vi "ATF Storage-RT_DAQ.vi"(8 "error in":errorcluster, 11 "Data FIFO Ref":T1) -> (0 "error out":errorcluster)   [LabVIEW 2022 SP3]
uses:
  RT Support/ATF Storage-RT_Global_R.vi
  RT Controls/ATF Storage-Data FIFO.ctl
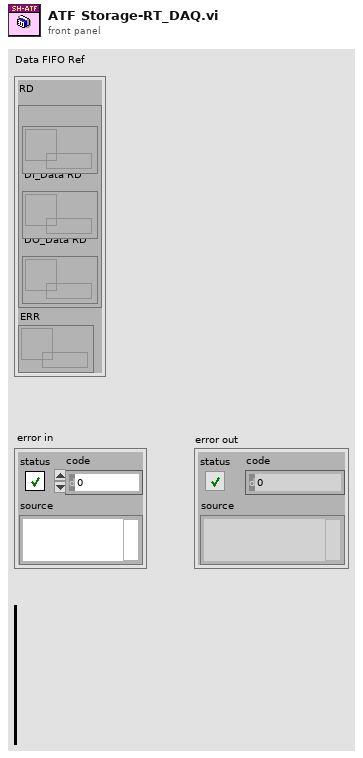
[diagram p1: front panel]
types:
  T1 = typedef "ATF Storage-Data FIFO.ctl" = cluster{"RD":cluster{"AI_V_Data RD":refnum<queue>, "DI_Data RD":refnum<queue>, "DO_Data RD":refnum<queue>}, "ERR":refnum<queue>}
  T2 = enum16{"Initialize", "Create Task", "Start", "Acquire", "Stop", "Exit"}
  T3 = cluster{"AI_Task":refnum<k21>, "AO_Task":refnum<k21>, "DI_Task":refnum<k21>, "DO_Task":refnum<k21>, "ACC_Task":refnum<k21>, "TC_Task":refnum<k21>, "AI_V_Task":refnum<k21>, " FIFO Ref":T1, "Config":cluster{"AO config":cluster{"Channel_Name":string, "Channel_Number":string, "Default_Value":dbl, "Units":string}[], "AI config":cluster{"Channel_Name":string, "Channel_Number":string, "Pre_Scale_min":dbl, "Pre_Scale_max":dbl, "Sensor_min":dbl, "Sensor_max":dbl, "Units":string}[], "DI config":cluster{"Channel_Name":string, "Channel_Number":string, "Default_Value":bool, "DI invert?":bool}[], "DO config":cluster{"Channel_Name":string, "Channel_Number":string, "Default_Value":bool, "DO invert?":bool}[], "TC config":cluster{"Channel_Name":string, "Channel_Number":string, "Pre_Scale_min":dbl, "Pre_Scale_max":dbl, "units":i32, " type":i32}[], "ACC config":cluster{"Channel_Name":string, "Channel_Number":string, "Pre_Scale_min":dbl, "Pre_Scale_max":dbl, "Terminal configuration":i32, "Sensitivity":dbl, "Sensitivity units":i32}[], "SG config":cluster{"Channel_Name":string, "Channel_Number":string, "Pre_Scale_min":dbl, "Pre_Scale_max":dbl}[], "Strain Gauge Settings":cluster{"poisson ratio":dbl, "nominal gage resistance":dbl, "gage factor":dbl}, "Bridge Settings":cluster{"voltage excitation value":dbl, "voltage excitation source":i32, "initial bridge voltage":dbl, "lead wire resistance":dbl, "strain configuration":i32}, "Sample Rate":cluster{"AI Sample Rate":dbl[], "AO Sample Rate":dbl[], "DI Sample Rate":dbl[], "TC Sample Rate":dbl[], "DO Sample Rate":dbl[], "SG Sample Rate":dbl[], "ACC Sample Rate":dbl[]}}}
  T4 = cluster{"Start DAQ":bool, "Stop DAQ":bool, "RT Stop":bool, "RT Exit":bool, "Start Seq":bool}
  T5 = cluster{"AO config":cluster{"Channel_Name":string, "Channel_Number":string, "Default_Value":dbl, "Units":string}[], "AI config":cluster{"Channel_Name":string, "Channel_Number":string, "Pre_Scale_min":dbl, "Pre_Scale_max":dbl, "Sensor_min":dbl, "Sensor_max":dbl, "Units":string}[], "DI config":cluster{"Channel_Name":string, "Channel_Number":string, "Default_Value":bool, "DI invert?":bool}[], "DO config":cluster{"Channel_Name":string, "Channel_Number":string, "Default_Value":bool, "DO invert?":bool}[], "TC config":cluster{"Channel_Name":string, "Channel_Number":string, "Pre_Scale_min":dbl, "Pre_Scale_max":dbl, "units":i32, "thermocouple type":i32}[], "ACC config":cluster{"Channel_Name":string, "Channel_Number":string, "Pre_Scale_min":dbl, "Pre_Scale_max":dbl, "Terminal configuration":i32, "Sensitivity":dbl, "Sensitivity units":i32}[], "SG config":cluster{"Channel_Name":string, "Channel_Number":string, "Pre_Scale_min":dbl, "Pre_Scale_max":dbl}[], "Strain Gauge Settings":cluster{"poisson ratio":dbl, "nominal gage resistance":dbl, "gage factor":dbl}, "Bridge Settings":cluster{"voltage excitation value":dbl, "voltage excitation source":i32, "initial bridge voltage":dbl, "lead wire resistance":dbl, "strain configuration":i32}, "Sample Rate":cluster{"AI Sample Rate":dbl[], "AO Sample Rate":dbl[], "DI Sample Rate":dbl[], "TC Sample Rate":dbl[], "DO Sample Rate":dbl[], "SG Sample Rate":dbl[], "ACC Sample Rate":dbl[]}}
  T6 = cluster{"Channel_Name":string, "Channel_Number":string, "Pre_Scale_min":dbl, "Pre_Scale_max":dbl, "Sensor_min":dbl, "Sensor_max":dbl, "Units":string}[]
  T7 = cluster{"Channel_Name":string, "Channel_Number":string, "Default_Value":bool, "DI invert?":bool}[]
  T8 = cluster{"Channel_Name":string, "Channel_Number":string, "Default_Value":bool, "DO invert?":bool}[]
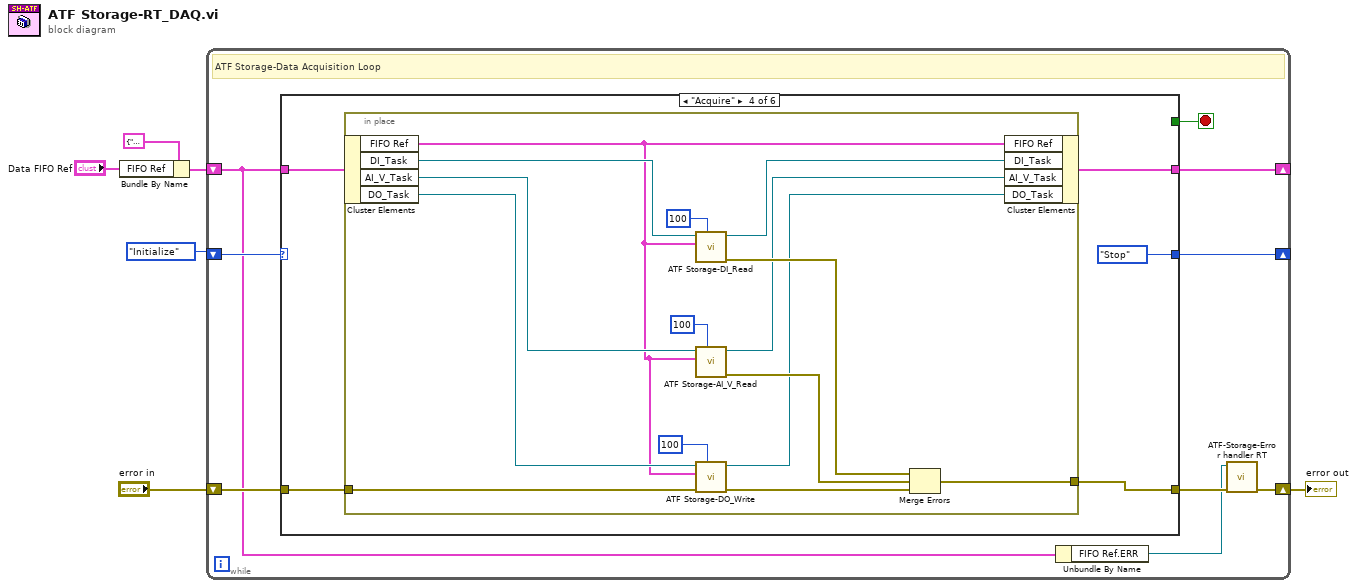
[diagram p0: block diagram]
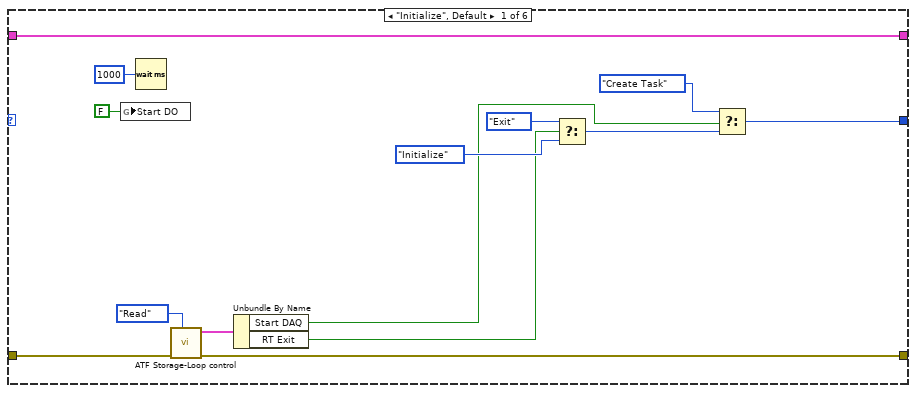
[diagram p2: hidden frame]
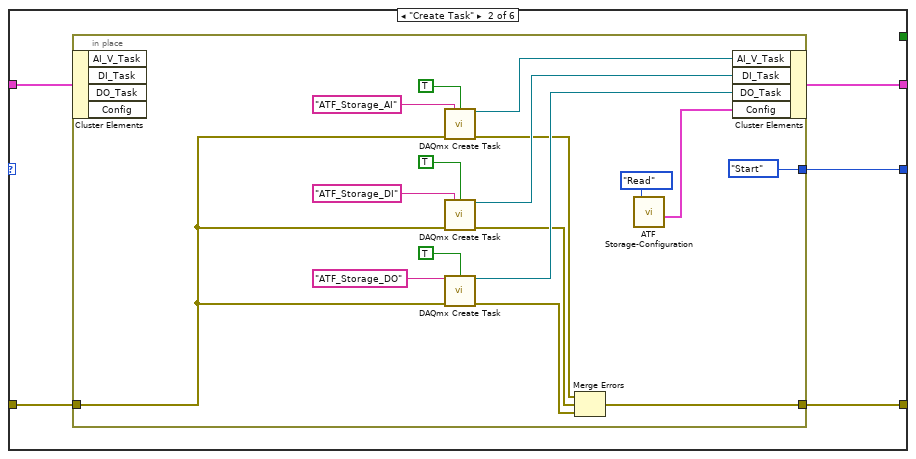
[diagram p3: hidden frame]
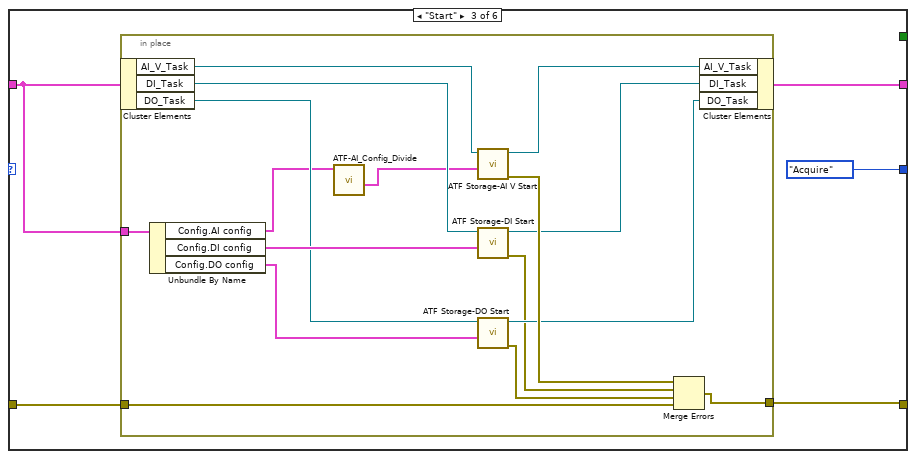
[diagram p4: hidden frame]
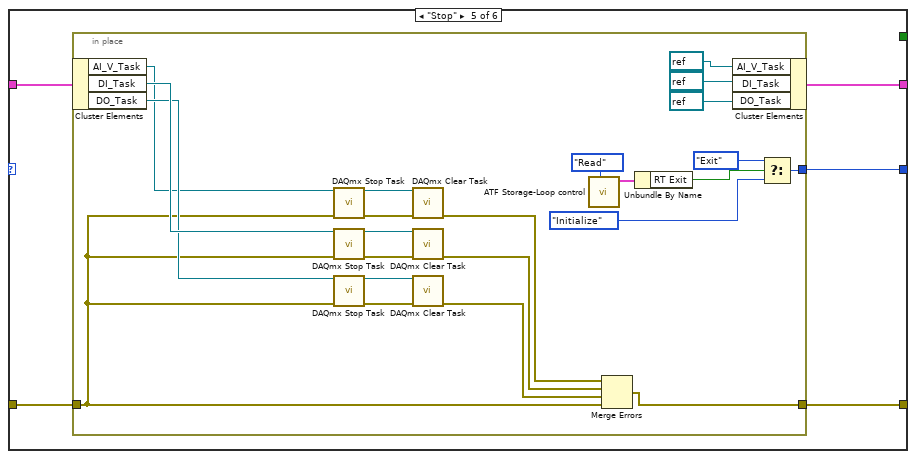
[diagram p5: hidden frame]
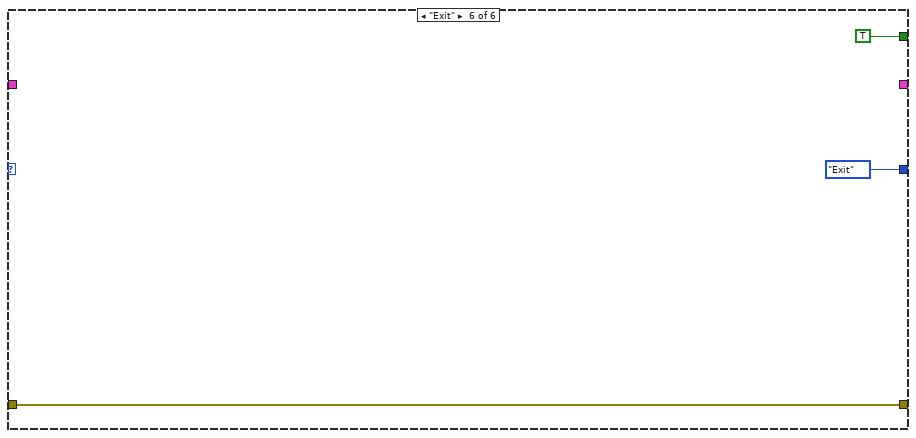
[diagram p6: hidden frame]
diagram:
  n1 = Bundle By Name(cluster=T3 {"AI_Task"="", "AO_Task"="", "DI_Task"="", "DO_Task"="", "ACC_Task"="", "TC_Task"="", "AI_V_Task"="", " FIFO Ref"={"RD"={"AI_V_Data RD"=refnum, "DI_Data RD"=refnum, "DO_Data RD"=refnum}, "ERR"=refnum}, "Config"={"AO config"=[], "AI config"=[], "DI config"=[], "DO config"=[], "TC config"=[], "ACC config"=[], "SG config"=[], "Strain Gauge Settings"={"poisson ratio"=0.0, "nominal gage resistance"=0.0, "gage factor"=0.0}, "Bridge Settings"={"voltage excitation value"=0.0, "voltage excitation source"=0, "initial bridge voltage"=0.0, "lead wire resistance"=0.0, "strain configuration"=0}, "Sample Rate"={"AI Sample Rate"=[], "AO Sample Rate"=[], "DI Sample Rate"=[], "TC Sample Rate"=[], "DO Sample Rate"=[], "SG Sample Rate"=[], "ACC Sample Rate"=[]}}}, "FIFO Ref"="Data FIFO Ref") -> (w1:T3)
  n2 = while {
    shift-right: [w13] -> _
    shift-left: T2."Initialize" -> [w15]
    shift-right: [w11] -> _
    shift-left: w1 -> [w7]
    shift-right: [w9] -> w5
    shift-left: "error in" -> [w14]
    stop <- w12 stop-if-true
    # "ATF Storage-Data Acquisition Loop"
    n3 = case shown="\"Acquire\"" w15 {
      tunnel: w14 -> [w19 w34 w56 w77 w95 w121]
      tunnel: [w18 w33 w55 w76 w96 w121] -> w10
      tunnel: [w28 w32 T2."Acquire" T2."Stop" w97 T2."Exit"] -> w13
      tunnel: w7 -> [w20 w31 w52 w75 w94 _]
      tunnel: [_ _ _ _ _ TRUE] -> w12
      tunnel: [w20 w30 w54 w74 w93 _] -> w11
      frame "Initialize", Default {
        n4 = global write "ATF Storage-RT_Global_R.vi" "Start DO"(FALSE ("Start DO")) -> ()
        n5 = Wait (ms)(milliseconds to wait=u32 1000) -> ()  [unwired: 1 out]
        n6 = call "ATF Storage-Loop control.vi"("Action"=enum16{"Init", "Write", "Read"}."Read", "error in (no error)"=w19) -> ("error Out"=w18:errorcluster, "Loop Control out"=w24:T4)  [unwired: 8 in]
        n7 = Unbundle By Name(w24) -> ("Start DAQ"=w23:bool, "RT Exit"=w22:bool)
        n8 = Select(t=T2."Exit", s=w22, f=T2."Initialize") -> (s? t:f=w25:T2)
        n9 = Select(t=T2."Create Task", s=w23, f=w25) -> (s? t:f=w28:T2)
      }
      frame "Create Task" {
        n10 = in-place "In Place Element Structure" {
          in-place-border: w34 -> [w40]
          in-place-border: [w49] -> w33
          in-place-border: [T2."Start"] -> w32
          n11 = in-place-cluster #1(w31) -> ()  [unwired: 4 out]
          n12 = call <vilib>:"DAQmx Create Task.vi"("new task name"="ATF_Storage_AI", "auto cleanup"=TRUE, "error in"=w40) -> ("task out"=w45:refnum<k21>, "error out"=w39:errorcluster)  [unwired: 11 in]
          n13 = call <vilib>:"DAQmx Create Task.vi"("new task name"="ATF_Storage_DI", "auto cleanup"=TRUE, "error in"=w40) -> ("task out"=w48:refnum<k21>, "error out"=w38:errorcluster)  [unwired: 11 in]
          n14 = call <vilib>:"DAQmx Create Task.vi"("new task name"="ATF_Storage_DO", "auto cleanup"=TRUE, "error in"=w40) -> ("task out"=w47:refnum<k21>, "error out"=w37:errorcluster)  [unwired: 11 in]
          n15 = Merge Errors(w39, w38, w37) -> (w49:errorcluster)
          n16 = call "ATF Storage-Configuration.vi"("Enum"=enum16{"Write", "Read"}."Read") -> ("Config out"=w35:T5)  [unwired: 10 in]
          n17 = in-place-cluster #1("AI_V_Task"=w45, "DI_Task"=w48, "DO_Task"=w47, "Config"=w35) -> (w30:T3)
        }
      }
      frame "Start" {
        n18 = in-place "In Place Element Structure" {
          in-place-border: w56 -> [w64]
          in-place-border: [w68] -> w55
          in-place-border: w52 -> [w62]
          n19 = in-place-cluster #2(w52) -> ("AI_V_Task"=w72:refnum<k21>, "DI_Task"=w67:refnum<k21>, "DO_Task"=w59:refnum<k21>)
          n20 = Unbundle By Name(w62) -> ("Config.AI config"=w58:T6, "Config.DI config"=w61:T7, "Config.DO config"=w60:T8)
          n21 = call "ATF-AI_Config_Divide.vi"("AI config"=w58) -> ("AI C"=w57:T6)  [unwired: 9 in, 1 out]
          n22 = call "ATF Storage-AI V Start.vi"("AI V"=w57, "Refnum in"=w72) -> ("error out"=w70:errorcluster, "Refnum out"=w71:refnum<k21>)  [unwired: 8 in]
          n23 = call "ATF Storage-DI Start.vi"("DI config"=w61, "Refnum in"=w67) -> ("error out"=w63:errorcluster, "Refnum out"=w66:refnum<k21>)  [unwired: 8 in]
          n24 = call "ATF Storage-DO Start.vi"("DO config"=w60, "Refnum in"=w59) -> ("error out"=w69:errorcluster, "Refnum out"=w65:refnum<k21>)  [unwired: 8 in]
          n25 = Merge Errors(w70, w63, w69, w64) -> (w68:errorcluster)
          n26 = in-place-cluster #2("AI_V_Task"=w71, "DI_Task"=w66, "DO_Task"=w65) -> (w54:T3)
        }
      }
      frame "Acquire" {
        n27 = in-place "In Place Element Structure" {
          in-place-border: w77 -> [w82]
          in-place-border: [w92] -> w76
          n28 = in-place-cluster #3(w75) -> ("FIFO Ref"=w78:T1, "DI_Task"=w84:refnum<k21>, "AI_V_Task"=w88:refnum<k21>, "DO_Task"=w89:refnum<k21>)
          n29 = call "ATF Storage-DI_Read.vi"("number of samples per channel"=100, "Data FIFO Ref"=w78, "DI_Task"=w84) -> ("error out"=w87:errorcluster, "task out"=w81:refnum<k21>)  [unwired: 7 in]
          n30 = call "ATF Storage-AI_V_Read.vi"("number of samples per channel"=100, "Data FIFO Ref"=w78, "AI_V_Task"=w88) -> ("error out"=w91:errorcluster, "AI_V_Task"=w80:refnum<k21>)  [unwired: 7 in]
          n31 = call "ATF Storage-DO_Write.vi"("Period"=i64 100, "error in (no error)"=w82, "Data FIFO Ref"=w78, "Refnum in"=w89) -> ("error out"=w90:errorcluster, "Refnum out"=w79:refnum<k21>)  [unwired: 6 in]
          n32 = Merge Errors(w87, w91, w90) -> (w92:errorcluster)
          n33 = in-place-cluster #3("FIFO Ref"=w78, "DI_Task"=w81, "AI_V_Task"=w80, "DO_Task"=w79) -> (w74:T3)
        }
      }
      frame "Stop" {
        n34 = in-place "In Place Element Structure" {
          in-place-border: [w118] -> w97
          in-place-border: [w115] -> w96
          in-place-border: w95 -> [w98]
          n35 = in-place-cluster #4(w94) -> ("AI_V_Task"=w108:refnum<k21>, "DI_Task"=w112:refnum<k21>, "DO_Task"=w111:refnum<k21>)
          n36 = call <vilib>:"DAQmx Stop Task.vi"("task/channels in"=w108, "error in"=w98) -> ("task out"=w107:refnum<k21>, "error out"=w106:errorcluster)  [unwired: 12 in]
          n37 = call <vilib>:"DAQmx Stop Task.vi"("task/channels in"=w112, "error in"=w98) -> ("task out"=w110:refnum<k21>, "error out"=w117:errorcluster)  [unwired: 12 in]
          n38 = call <vilib>:"DAQmx Stop Task.vi"("task/channels in"=w111, "error in"=w98) -> ("task out"=w109:refnum<k21>, "error out"=w116:errorcluster)  [unwired: 12 in]
          n39 = call <vilib>:"DAQmx Clear Task.vi"("task in"=w107, "error in"=w106) -> ("error out"=w105:errorcluster)  [unwired: 13 in]
          n40 = call <vilib>:"DAQmx Clear Task.vi"("task in"=w110, "error in"=w117) -> ("error out"=w114:errorcluster)  [unwired: 13 in]
          n41 = call <vilib>:"DAQmx Clear Task.vi"("task in"=w109, "error in"=w116) -> ("error out"=w113:errorcluster)  [unwired: 13 in]
          n42 = call "ATF Storage-Loop control.vi"("Action"=enum16{"Init", "Write", "Read"}."Read") -> ("Loop Control out"=w104:T4)  [unwired: 9 in, 1 out]
          n43 = Merge Errors(w105, w114, w113, w98) -> (w115:errorcluster)
          n44 = Unbundle By Name(w104) -> ("RT Exit"=w103:bool)
          n45 = in-place-cluster #4("AI_V_Task"=refnum<k21> refnum, "DI_Task"=refnum<k21> refnum, "DO_Task"=refnum<k21> refnum) -> (w93:T3)
          n46 = Select(t=T2."Exit", s=w103, f=T2."Initialize") -> (s? t:f=w118:T2)
        }
      }
      frame "Exit" {
      }
    }
    n47 = Unbundle By Name(w7) -> ("FIFO Ref.ERR"=w8:refnum<queue>)
    n48 = call "ATF-Storage-Error handler RT.vi"("error in"=w10, "Message Queue"=w8) -> ("error out"=w9:errorcluster)  [unwired: 8 in, 1 out]
  }
  "error out" <- w5
